vi "niScope Actual Meas Wfm Size.vi"(8 "error in":errorcluster, 10 "arrayMeasFunction":i32, 11 "instrument handle":refnum<k15>) -> (0 "error out":errorcluster, 2 "meas wfm size":i32, 3 "instrument handle out":refnum<k15>)   [LabVIEW 2013]
doc: "Returns the total available size of an array measurement acquisition in samples."
uses:
  niScope_32.dll
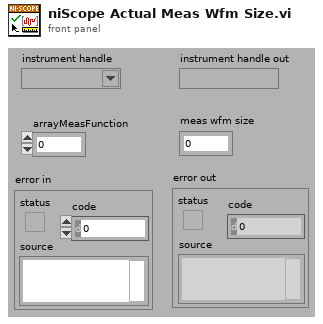
[diagram p1: front panel]
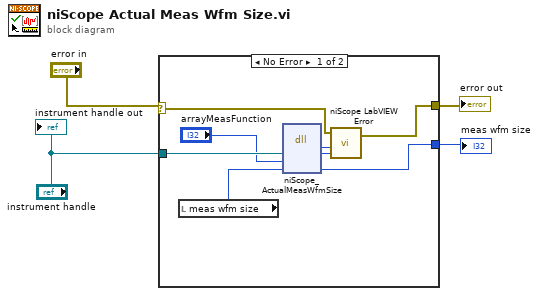
[diagram p0: block diagram]
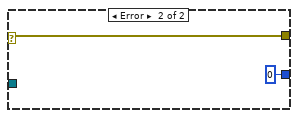
[diagram p2: hidden frame]
diagram:
  n1 = case shown="No Error" "error in" {
    selector: "error in" -> [w5 w13]
    tunnel: [w10 w13] -> w4
    tunnel: [w7 0 ("numWaveforms")] -> w3
    tunnel: "instrument handle" -> [w9 _]
    frame No Error {
      n2 = local read "meas wfm size"() -> (w8:i32)
      n3 = dll-call lib="niScope_*.*" fn="niScope_ActualMeasWfmSize"("instrument handle"=w9, "arrayMeasFunction"="arrayMeasFunction", "measWfmSize"=w8) -> ("status"=w12:i32, "instrument handle"=w11:u32, "measWfmSize"=w7:i32)  [unwired: 4 in, 2 out]
      n4 = call <instrlib>:"niScope LabVIEW Error.vi"("instrument handle"=w11, "niScope error code (0)"=w12, "error in (no error)"=w5) -> ("error out"=w10:errorcluster)  [unwired: 2 in]
    }
    frame Error {
    }
  }
  "meas wfm size" <- w3
  "error out" <- w4
  "instrument handle out" <- "instrument handle"
